vi "AuMT8852B Initial Carrier Results Query.vi"(8 "error in (no error)":errorcluster, 11 "VISA session":refnum<visa-resource-name>) -> (0 "error out":errorcluster, 2 "error code":i32, 3 "VISA session out":refnum<visa-resource-name>, 4 "Results":T1 {"Max negative offset (kHz)" format="%.2f"; "Max positive offset (kHz)" format="%.2f"; "Test average offset (kHz)" format="%.2f"; "Frequency offset (kHz)" format="%.2f"})   [LabVIEW 2017]
doc: "Anritsu MT8852B Bluetooth Tester\n\nReturns the results of the Initial Carrier test.\n\nOUTPUTS\nResults - measurements made during the test."
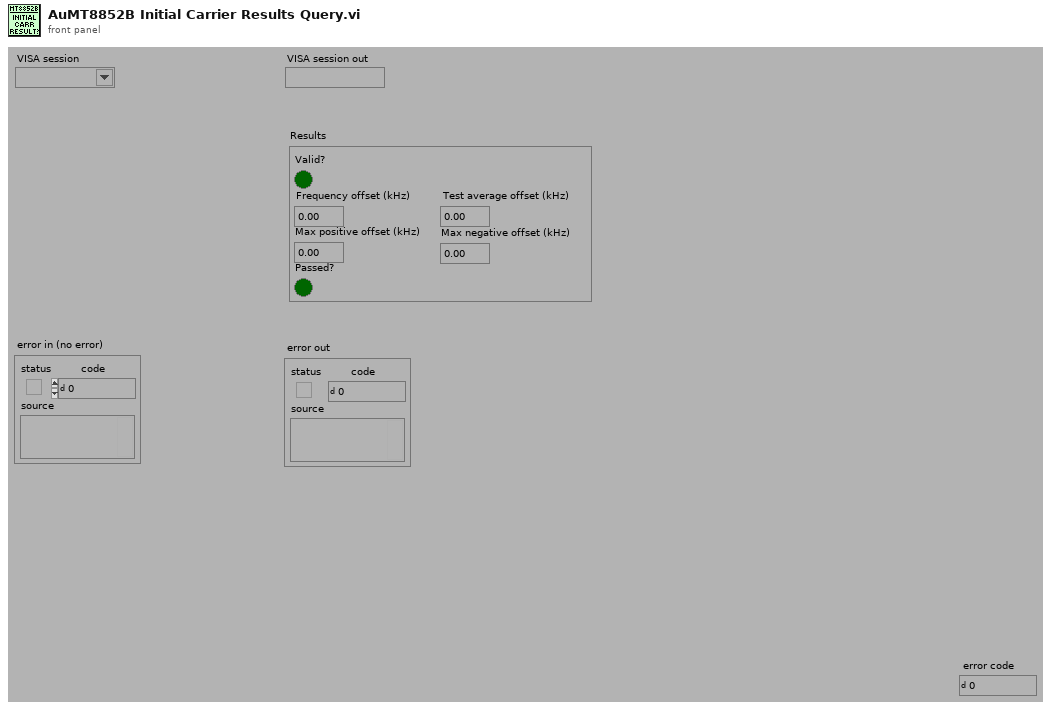
[diagram p1: front panel]
types:
  T1 = cluster{"Valid?":bool, "Frequency offset (kHz)":dbl, "Test average offset (kHz)":dbl, "Max positive offset (kHz)":dbl, "Max negative offset (kHz)":dbl, "Passed?":bool}
  T2 = enum16{"Simulate", "Range check", "Cache", "Query instrument status"}
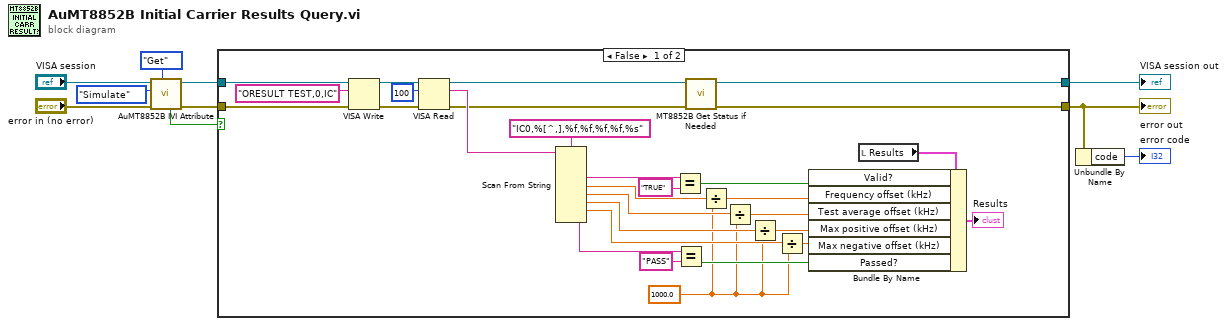
[diagram p0: block diagram]
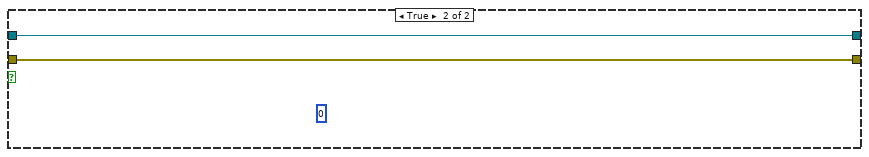
[diagram p2: hidden frame]
diagram:
  n1 = call <instrlib>:"AuMT8852B IVI Attribute.vi"("Set/Get (Set)"=enum16{"Set", "Get"}."Get", "error in (no error)"="error in (no error)", "Flag (Simulate)"=T2."Simulate", "VISA session"="VISA session") -> ("error out"=w7:errorcluster, "VISA session out"=w9:refnum<visa-resource-name>, "Value out"=w3:bool)  [unwired: 5 in]
  n2 = case shown="False" w3 {
    tunnel: [w26 w41] -> w10
    tunnel: [w25 w40] -> w1
    tunnel: w9 -> [w38 w41]
    tunnel: w7 -> [w37 w40]
    frame False {
      w11 = 1000.0 ("y")
      n3 = VISA Write(VISA resource name=w38, write buffer="ORESULT TEST,0,IC" ("write buffer (\"\")"), error in (no error)=w37) -> (VISA resource name out=w36:refnum<visa-resource-name>, error out=w35:errorcluster)  [unwired: 1 out]
      n4 = VISA Read(VISA resource name=w36, byte count=u32 100 ("byte count (0)"), error in (no error)=w35) -> (VISA resource name out=w23:refnum<visa-resource-name>, read buffer=w24:string, error out=w22:errorcluster)  [unwired: 1 out]
      n5 = Scan From String(format string="IC0,%[^,],%f,%f,%f,%f,%s" ("Format String"), input string=w24) -> (output 1=w30:string, output 2=w19:dbl, output 3=w16:dbl, output 4=w14:dbl, output 5=w12:dbl, output 6=w20:string)  [unwired: 8 in, 3 out]
      n6 = Equal?(x=w30, y="TRUE") -> (x = y?=w31:bool)
      n7 = Equal?(x=w20, y="PASS") -> (x = y?=w21:bool)
      n8 = call <instrlib>:"MT8852B Get Status if Needed.vi"("error in (no error)"=w22, "VISA session"=w23) -> ("error out"=w25:errorcluster, "VISA session out"=w26:refnum<visa-resource-name>)  [unwired: 8 in]
      n9 = Divide(x=w19, y=w11) -> (x/y=w15:dbl)
      n10 = Divide(x=w16, y=w11) -> (x/y=w18:dbl)
      n11 = Divide(x=w14, y=w11) -> (x/y=w17:dbl)
      n12 = Divide(x=w12, y=w11) -> (x/y=w13:dbl)
      n13 = local read "Results"() -> (w32:T1)
      n14 = Bundle By Name(cluster=w32, "Valid?"=w31, "Frequency offset (kHz)"=w15, "Test average offset (kHz)"=w18, "Max positive offset (kHz)"=w17, "Max negative offset (kHz)"=w13, "Passed?"=w21) -> (→"Results":T1)
    }
    frame True {
      (unwired) u8 0
    }
  }
  "error out" <- w1
  "VISA session out" <- w10
  n15 = Unbundle By Name(w1) -> ("code"=→"error code":i32)
